vi "Build Result Array from Shots.vi"(7 "Analysis Selections":T1[](array[typedef]), 8 "Injection Event Dwell Period (ms)":dbl, 10 "Injection Event Count":u32, 11 "Shot Info Array":T2[](array[typedef]) {"Results"."Off-Stage Avg Current" format="%#.6g"; "Results"."Total Voltage Pulses" format="%#.6g"; "Results"."Off-Stage Min Current" format="%#.6g"; "Results"."Off-Stage Max Current" format="%#.6g"}) -> (1 "Result Array":dbl[](array[numeric]))   [LabVIEW 2015, in "Fuel Injection Addon Engine.lvlib"]
uses:
  Fuel Injection Addon Engine.lvlib
  RT Analysis/Controls/Shot Information Control.ctl
  Types/Stage.Measurements.ctl
  Shared/Types/Analysis.Channels.Select.ctl
  Shared/Fuel Injection Addon Shared.lvlib
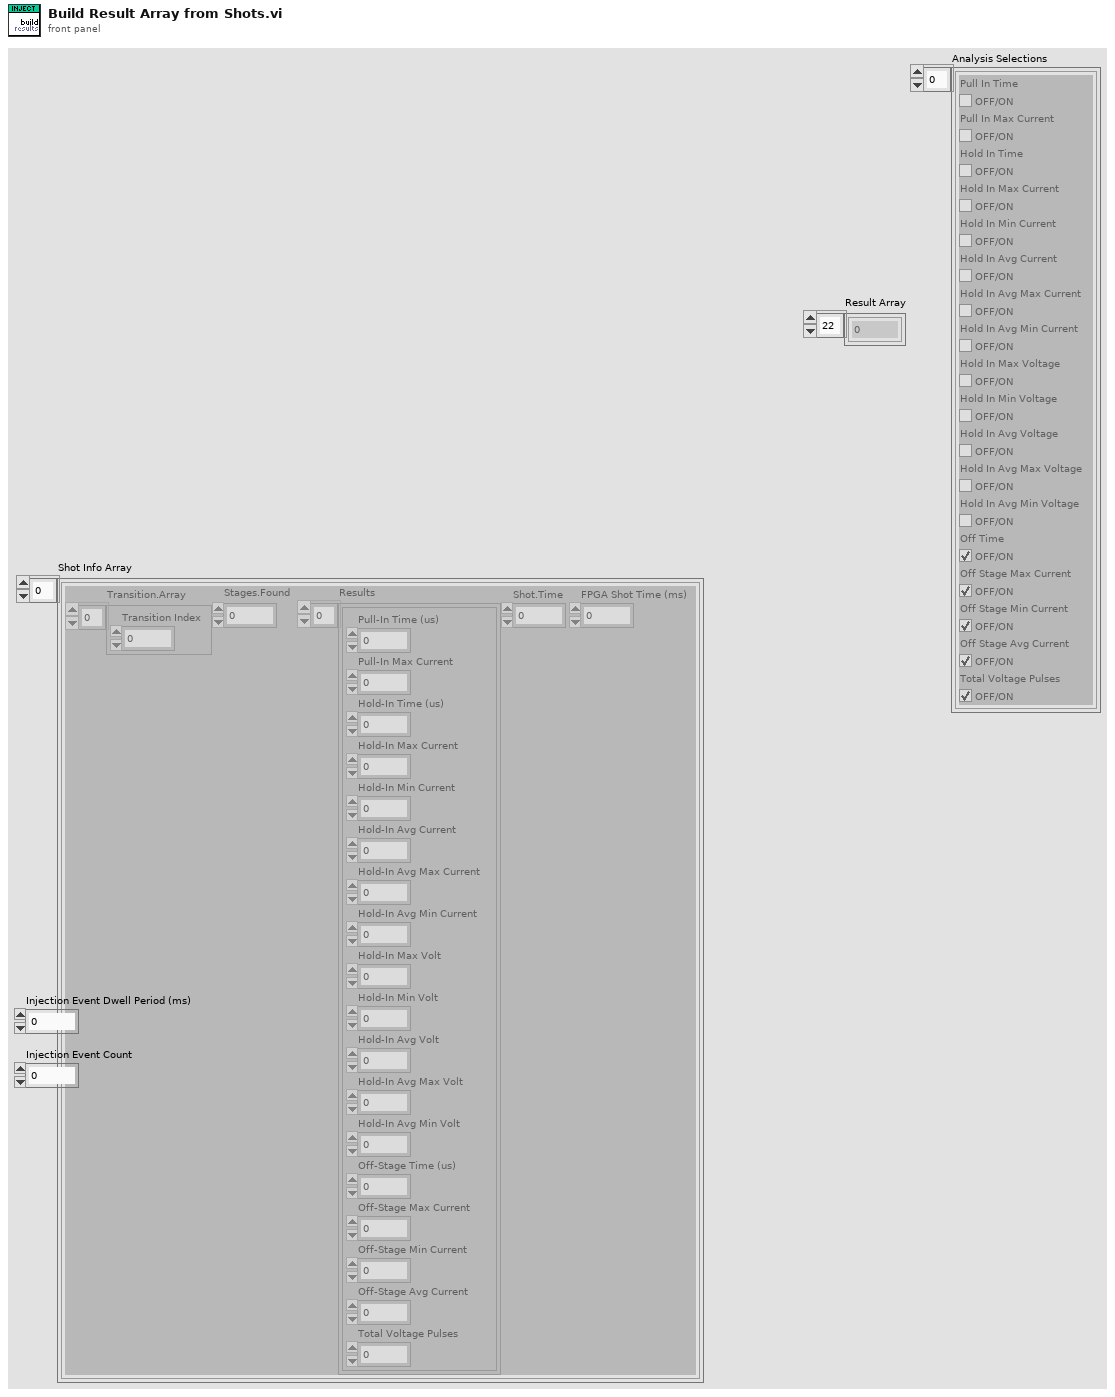
[diagram p1: front panel]
types:
  T1 = typedef "Fuel Injection Addon Shared.lvlib/Analysis.Channels.Select.ctl" = cluster{"Pull In Time":bool, "Pull In Max Current":bool, "Hold In Time":bool, "Hold In Max Current":bool, "Hold In Min Current":bool, "Hold In Avg Current":bool, "Hold In Avg Max Current":bool, "Hold In Avg Min Current":bool, "Hold In Max Voltage":bool, "Hold In Min Voltage":bool, "Hold In Avg Voltage":bool, "Hold In Avg Max Voltage":bool, "Hold In Avg Min Voltage":bool, "Off Time":bool, "Off Stage Max Current":bool, "Off Stage Min Current":bool, "Off Stage Avg Current":bool, "Total Voltage Pulses":bool}
  T2 = typedef "Fuel Injection Addon Engine.lvlib/Shot Information Control.ctl" = cluster{"Transition.Array":i32[], "Stages.Found":u16, "Results":T3[], "Shot.Time":dbl, "FPGA Shot Time (ms)":dbl}
  T3 = typedef "Fuel Injection Addon Engine.lvlib/Stage.Measurements.ctl" = cluster{"Pull-In Time (us)":dbl, "Pull-In Max Current":dbl, "Hold-In Time (us)":dbl, "Hold-In Max Current":dbl, "Hold-In Min Current":dbl, "Hold-In Avg Current":dbl, "Hold-In Avg Max Current":dbl, "Hold-In Avg Min Current":dbl, "Hold-In Max Volt":dbl, "Hold-In Min Volt":dbl, "Hold-In Avg Volt":dbl, "Hold-In Avg Max Volt":dbl, "Hold-In Avg Min Volt":dbl, "Off-Stage Time (us)":dbl, "Off-Stage Max Current":dbl, "Off-Stage Min Current":dbl, "Off-Stage Avg Current":dbl, "Total Voltage Pulses":dbl}
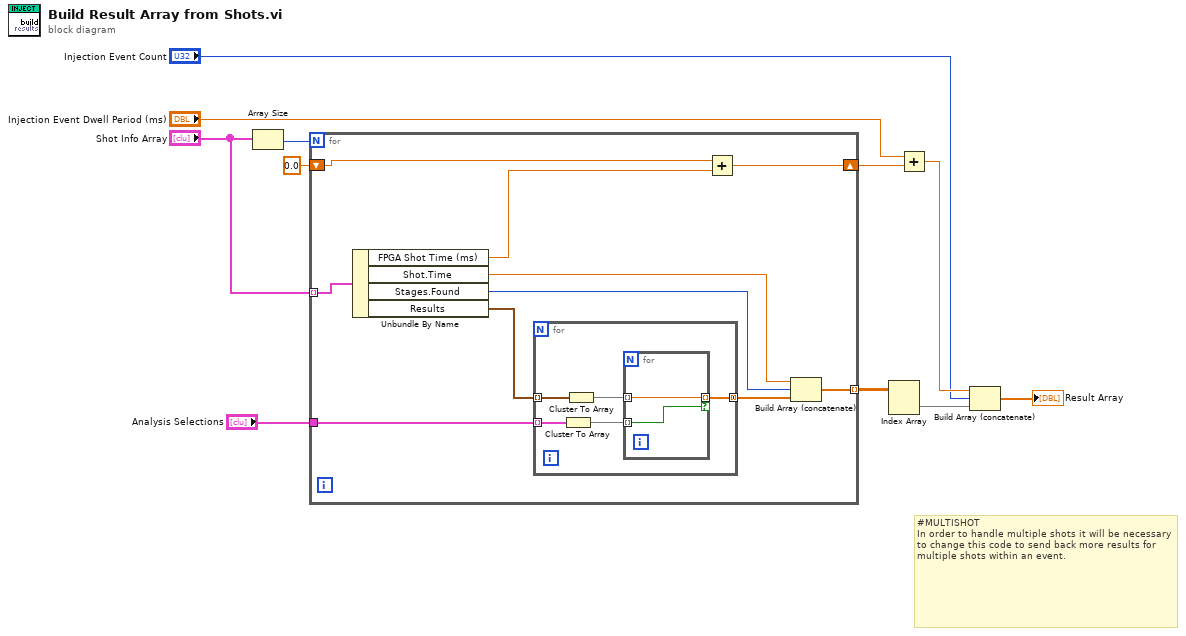
[diagram p0: block diagram]
diagram:
  # "#MULTISHOT\nIn order to handle multiple shots it will be necessary to change this code to send back more results for multiple shots within an event."
  n1 = Array Size(array="Shot Info Array") -> (size(s)=w6:i32)
  n2 = for {
    N: w6 -> [_]
    tunnel: "Shot Info Array" -> [w21] mode=indexing
    shift-right: [w20] -> w8
    shift-left: 0.0 -> [w19]
    tunnel: [w15] -> w10 mode=indexing
    tunnel: "Analysis Selections" -> [w17]
    n3 = Unbundle By Name(w21) -> ("FPGA Shot Time (ms)"=w12:dbl, "Shot.Time"=w16:dbl, "Stages.Found"=w13:u16, "Results"=w18:T3[])
    n4 = for {
      tunnel: w18 -> [w25] mode=indexing
      tunnel: w17 -> [w26] mode=indexing
      tunnel: [w22] -> w14 mode=concatenating
      n5 = Cluster To Array(cluster=w26) -> (array=w23:bool[])
      n6 = Cluster To Array(cluster=w25) -> (array=w24:dbl[])
      n7 = for {
        tunnel: w24 -> [w28] mode=indexing
        tunnel: w23 -> [w27] mode=indexing
        tunnel: [w28] -> w22 mode=indexing if=w27
      }
    }
    n8 = Add(x=w19, y=w12) -> (x+y=w20:dbl)
    n9 = Build Array (concatenate)(w16, w13, w14) -> (w15:dbl[])
  }
  n10 = Index Array(array=w10) -> (element=w11:dbl[])  [unwired: 2 in]
  n11 = Add(x="Injection Event Dwell Period (ms)", y=w8) -> (x+y=w9:dbl)
  n12 = Build Array (concatenate)(w9, "Injection Event Count", w11) -> (→"Result Array":dbl[])
